vi "Add Item.vi"(6 "Data":variant, 8 "error in (no error)":errorcluster, 9 "Text":string, 10 "Parent Tag":refnum<class "Tree Tag Class.lvclass">, 11 "Tree_LVOOP in":refnum<class "Tree Class.lvclass">) -> (0 "error out":errorcluster, 2 "Upmost Created Tag":refnum<class "Tree Tag Class.lvclass">, 3 "Tree_LVOOP out":refnum<class "Tree Class.lvclass">)   [LabVIEW 2012, in "Tree Tools.lvlib" / "Tree Class.lvclass"]
uses:
  Tree Class.lvclass
  Tree Tag Class/Tree Tag Class.lvclass
  Tree Class.lvclass/Tree Class.ctl
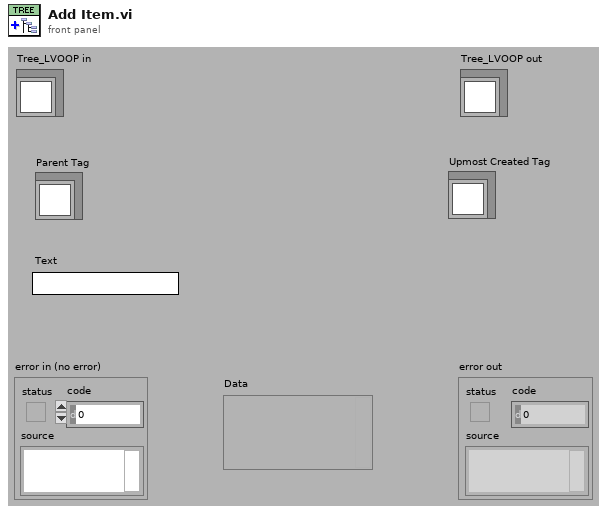
[diagram p1: front panel]
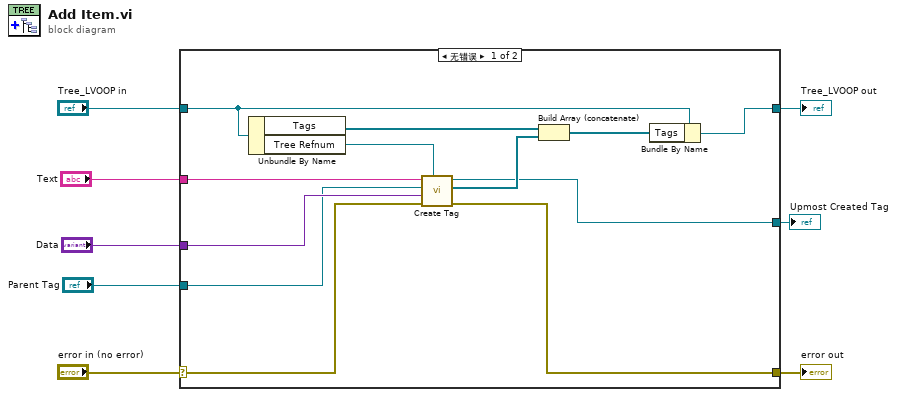
[diagram p0: block diagram]
diagram:
  n1 = case shown="无错误" "error in (no error)" {
    selector: "error in (no error)" -> [w10 w22]
    tunnel: [w9 w22] -> w7
    tunnel: [w16 w21] -> w5
    tunnel: "Tree_LVOOP in" -> [w17 w21]
    tunnel: "Text" -> [w20 _]
    tunnel: "Data" -> [w18 _]
    tunnel: "Parent Tag" -> [w13 _]
    tunnel: [w11 _] -> w1
    frame No Error {
      n2 = Unbundle By Name(w17) -> ("Tags"=w15:refnum<class "Tree Tag Class.lvclass">[], "Tree Refnum"=w19:refnum<vi>)
      n3 = call "Create Tag.vi"("OwnerTree (if Parent empty)"=w19, "error in (no error)"=w10, "Data"=w18, "Parent Tag"=w13, "Text"=w20) -> ("error out"=w9:errorcluster, "Created Tags"=w12:refnum<class "Tree Tag Class.lvclass">[], "Tag_LVOOP out"=w11:refnum<class "Tree Tag Class.lvclass">)  [unwired: 4 out]
      n4 = Build Array (concatenate)(w15, w12) -> (w14:refnum<class "Tree Tag Class.lvclass">[])
      n5 = Bundle By Name(cluster=w17, "Tags"=w14) -> (w16:refnum<class "Tree Class.lvclass">)
    }
    frame Error {
    }
  }
  "error out" <- w7
  "Tree_LVOOP out" <- w5
  "Upmost Created Tag" <- w1
